vi "MICS Power UI.vi"() -> ()   [LabVIEW 2010]
panel:
  in  "Number of \"Open Session\" Retry Attempts (3)":i32=3
  in  "245TX_Power":i8=6
  in  "MICS inputs":T1={"address"="COM5", "chan"=2, "ID"=4412} {"ID" format="%04x"; "chan" min=1 max=10 step=1}
  in  "Samples":i32=10
  in  "MICS Power Range":cluster{"Min":dbl, "Max":dbl, "Increment":dbl}={"Min"=10.0, "Max"=25.0, "Increment"=1.0}
  in  "Attenuation dB (0)":dbl
  out "error out":errorcluster
  out "Percent Successful vs. MICS Power":cluster{dbl, dbl}[](graph)
  in  "stop":bool
  in  "error in (no error)":errorcluster
  # "Acceptable values are 0x00\nthrough 0x3F, inclusive."
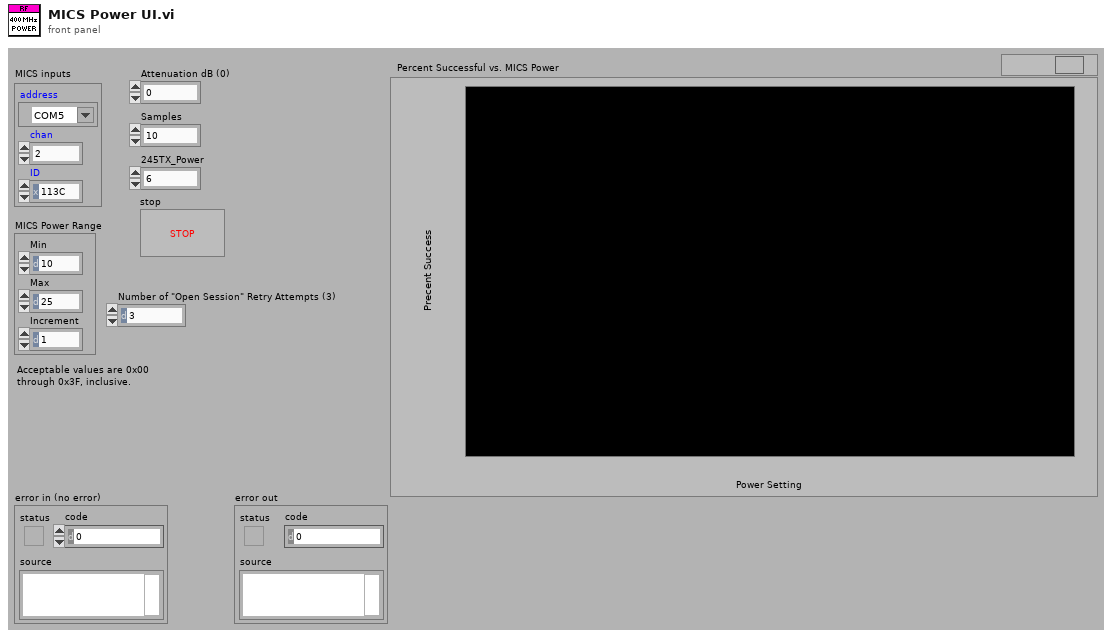
[diagram p1: front panel]
types:
  T1 = cluster{"address":refnum<visa-resource-name>, "chan":u16, "ID":u32}
  T2 = cluster{"ConfigFlags":u8, "ImplantID":u32, "CompanyID":u8, "Normal_Comm":cluster{"RF_Channel":u8, "UserData":u8, "TX_Mod":u8, "RX_Mod":u8, "RX_BlockSize":u8, "BlockPerPack":u8, "TX_BlockSize":u8}, "Emerg_Comm":cluster{"RF_Channel":u8, "UserData":u8, "TX_Mod":u8, "RX_Mod":u8, "TX_BlockSize":u8, "BlockPerPack":u8, "RX_BlockSize":u8}, "ImplantRev":u8, "245TX_PowerCal":i8, "245TX_Power":i8, "CCA_RSSI_Thresholds":cluster{"ch0":u16, "ch1":u16, "ch2":u16, "ch3":u16, "ch4":u16, "ch5":u16, "ch6":u16, "ch7":u16, "ch8":u16, "ch9":u16}}
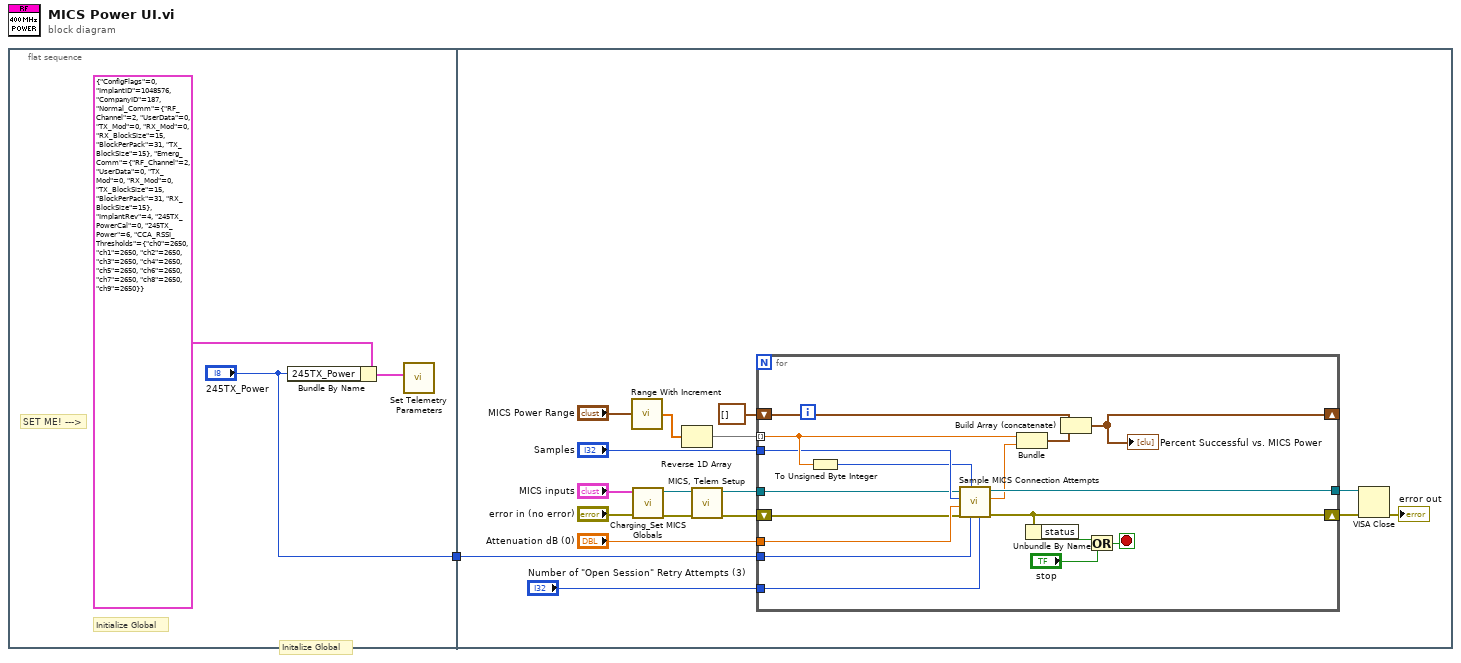
[diagram p0: block diagram]
diagram:
  n1 = flat-sequence {
    tunnel: ["245TX_Power"] -> w1
    tunnel: w1 -> [w6]
    frame #0 {
      # "Initialize Global"
      # "SET ME! --->"
      # "Initalize Global"
      n2 = Bundle By Name(cluster=T2 {"ConfigFlags"=0, "ImplantID"=1048576, "CompanyID"=187, "Normal_Comm"={"RF_Channel"=2, "UserData"=0, "TX_Mod"=0, "RX_Mod"=0, "RX_BlockSize"=15, "BlockPerPack"=31, "TX_BlockSize"=15}, "Emerg_Comm"={"RF_Channel"=2, "UserData"=0, "TX_Mod"=0, "RX_Mod"=0, "TX_BlockSize"=15, "BlockPerPack"=31, "RX_BlockSize"=15}, "ImplantRev"=4, "245TX_PowerCal"=0, "245TX_Power"=6, "CCA_RSSI_Thresholds"={"ch0"=2650, "ch1"=2650, "ch2"=2650, "ch3"=2650, "ch4"=2650, "ch5"=2650, "ch6"=2650, "ch7"=2650, "ch8"=2650, "ch9"=2650}} ("MICS_Config_In"), "245TX_Power"="245TX_Power") -> (w3:T2)
      n3 = call "Set Telemetry Parameters.vi"("MICS_Config_In"=w3) -> ()  [unwired: 11 in]
    }
    frame #1 {
      n4 = call "Range With Increment.vi"("Range"="MICS Power Range") -> ("Output Array"=w16:dbl[])
      n5 = call "Charging_Set MICS Globals.vi"("error in"="error in (no error)", "MICS inputs"="MICS inputs") -> ("error out"=w9:errorcluster, "address"=w11:refnum<visa-resource-name>)  [unwired: 4 in]
      n6 = Reverse 1D Array(array=w16) -> (reversed array=w13:dbl[])
      n7 = call "MICS, Telem Setup.vi"("error in"=w9, "VISA resource"=w11) -> ("error out"=w8:errorcluster, "VISA resource dup"=w7:refnum<visa-resource-name>)  [unwired: 8 in]
      n8 = for {
        shift-right: [w36] -> _
        shift-left: cluster{dbl, dbl}[] [] ("XY Graph") -> [w38]
        tunnel: [w35] -> w20
        tunnel: w13 -> [w29] mode=indexing
        tunnel: "Samples" -> [w28]
        tunnel: "Attenuation dB (0)" -> [w27]
        tunnel: w7 -> [w24]
        shift-right: [w34] -> w19
        shift-left: w8 -> [w25]
        tunnel: w6 -> [w23]
        tunnel: "Number of \"Open Session\" Retry Attempts (3)" -> [w22]
        stop <- w32 stop-if-true
        n9 = To Unsigned Byte Integer(number=w29) -> (unsigned 8bit integer=w26:u8)
        n10 = call "Sample MICS Connection Attempts.vi"("Number of \"Open Session\" Retry Attempts (3)"=w22, "2.45 GHz Wake-Up Power"=w23, "400 MHz MICS Power Setting"=w26, "error in"=w25, "Attenuation dB"=w27, "Samples (1)"=w28, "MICS Resource Name"=w24) -> ("error out"=w34:errorcluster, "Percent Successful"=w30:dbl, "MICS Resource Name out"=w35:refnum<visa-resource-name>)  [unwired: 1 in, 1 out]
        n11 = Bundle(w29, "Percent Successful"=w30) -> (w37:cluster{dbl, "Percent Successful":dbl})  [unwired: 1 in]
        n12 = Unbundle By Name(w34) -> ("status"=w33:bool)
        n13 = Build Array (concatenate)(w38, w37) -> (w36:cluster{dbl, "Percent Successful":dbl}[])
        "Percent Successful vs. MICS Power" <- w36
        n14 = Or(x=w33, y="stop") -> (x .or. y?=w32:bool)
      }
      n15 = VISA Close(VISA resource name=w20, error in (no error)=w19) -> (error out=→"error out":errorcluster)
    }
  }
